vi "ClassicEventDrivenVI.vi"() -> ()   [LabVIEW 2014]
panel:
  in  "stop":bool
  out "What happened?":string
  in  "Button 2":bool
  in  "Button 1":bool
  in  "Numeric":dbl
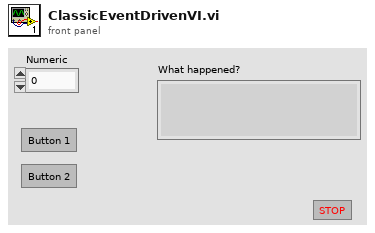
[diagram p1: front panel]
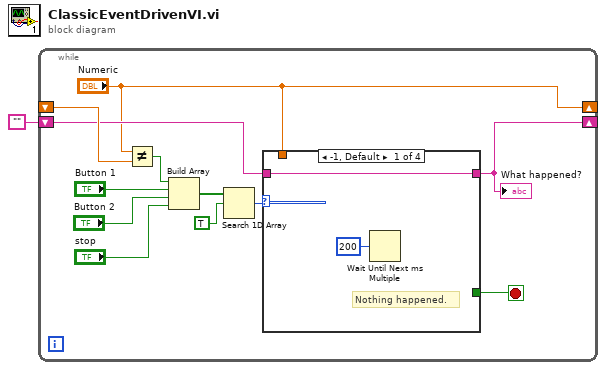
[diagram p0: block diagram]
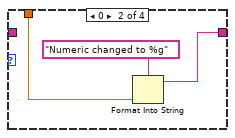
[diagram p2: hidden frame]
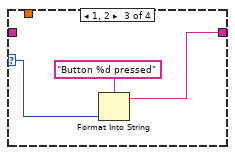
[diagram p3: hidden frame]
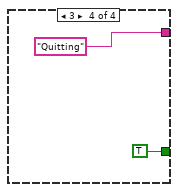
[diagram p4: hidden frame]
diagram:
  n1 = while {
    shift-right: ["Numeric"] -> _
    shift-left: _ -> [w13]
    shift-right: [w5] -> _
    shift-left: "" -> [w6]
    stop <- w3 stop-if-true
    n2 = Not Equal?(x="Numeric", y=w13) -> (x != y?=w12:bool)
    n3 = Build Array(w12, "Button 1", "Button 2", "stop") -> (w7:bool[])
    n4 = Search 1D Array(1D array=w7, element=TRUE) -> (index of element=w8:i32)  [unwired: 1 in]
    n5 = case shown="-1, Default" w8 {
      selector: w8 -> [_ _ w20 _]
      tunnel: w6 -> [w15 _ _ _]
      tunnel: [w15 w16 w19 "Quitting"] -> w5
      tunnel: "Numeric" -> [_ w18 _ _]
      tunnel: [_ _ _ TRUE] -> w3
      frame -1, Default {
        # "Nothing happened."
        n6 = Wait Until Next ms Multiple(millisecond multiple=u32 200) -> ()  [unwired: 1 out]
      }
      frame 0 {
        n7 = Format Into String(format string="Numeric changed to %g", w18) -> (resulting string=w16:string)  [unwired: 2 in, 1 out]
      }
      frame 1, 2 {
        n8 = Format Into String(format string="Button %d pressed", w20) -> (resulting string=w19:string)  [unwired: 2 in, 1 out]
      }
      frame 3 {
      }
    }
    "What happened?" <- w5
  }
